vi "Filter Ancestor Names.vi"(8 "error in (no error)":errorcluster, 9 "Name":string, 10 "Start Index":i32, 11 "Config Manager in":refnum<class "Config Manager.lvclass">) -> (0 "error out":errorcluster, 2 "Elements":refnum<class "Config Element.lvclass">[](array[class]), 3 "Config Manager out":refnum<class "Config Manager.lvclass">)   [LabVIEW 2020, in "CDM-Config.lvlib" / "Config Manager.lvclass"]
uses:
  Config Manager.lvclass
  Config Element/Config Element.lvclass
panel:
  out "Array":T1(array[cluster])
  out "delimited string":string
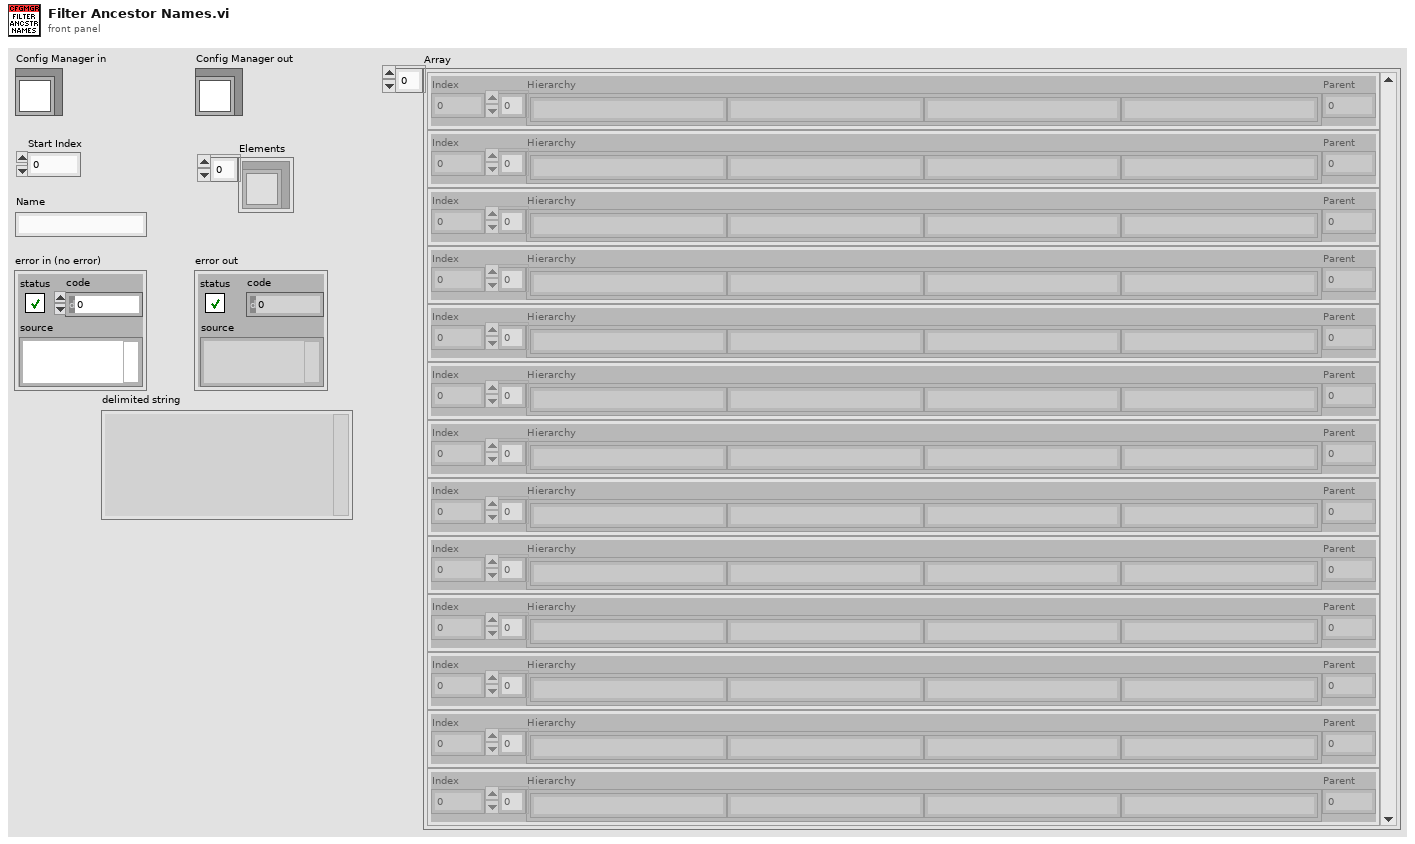
[diagram p1: front panel]
types:
  T1 = cluster{"Index":i32, "Hierarchy":string[], "Parent":i32}[]
  T2 = typedef "CDM-Config.lvlib/Config Manager.lvclass/Ref Data.ctl" = cluster{"Elements":refnum<class "Config Element.lvclass">[], "Hierarchy Map":map{string[], i32}, "Element Map":map{refnum<class "Config Element.lvclass">, i32}}
  T3 = cluster{"Index":i32, "Hierarchy":string[], "Index":i32}
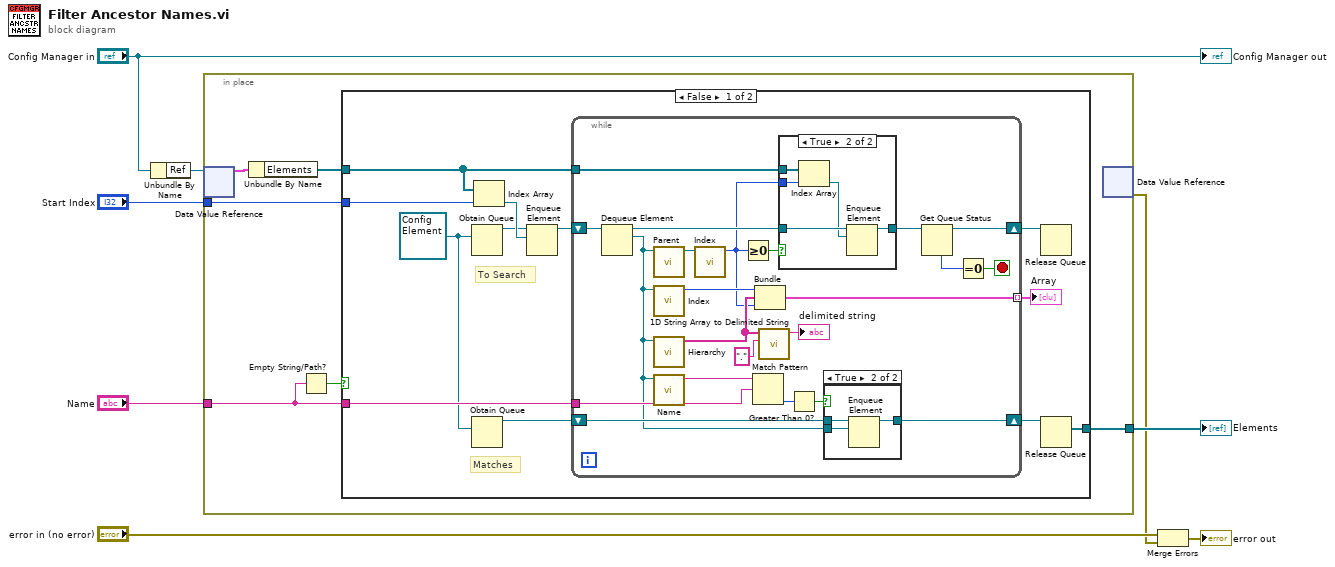
[diagram p0: block diagram]
diagram:
  n1 = Unbundle By Name("Config Manager in") -> ("Ref"=w6:refnum<data-value>)
  n2 = in-place {
    in-place-border: "Start Index" -> [w12]
    in-place-border: "Name" -> [w10]
    in-place-border: [w11] -> w2
    n3 = in-place-dvr #1(w6) -> (w14:T2)  [unwired: 1 out]
    n4 = Unbundle By Name(w14) -> ("Elements"=w13:refnum<class "Config Element.lvclass">[])
    n5 = Empty String/Path?(string/path=w10) -> (empty?=w9:bool)
    n6 = case shown="False" w9 {
      tunnel: w13 -> [w26 w59]
      tunnel: w12 -> [w25 _]
      tunnel: w10 -> [w22 _]
      tunnel: [w16 w59] -> w11
      frame False {
        w21 = refnum<class "Config Element.lvclass"> refnum ("CDM-Config.lvlib:Config Element.lvclass")
        # "Matches"
        # "To Search"
        n7 = Obtain Queue(element data type=w21) -> (queue out=w20:refnum<queue>)  [unwired: 4 in, 2 out]
        n8 = Obtain Queue(element data type=w21) -> (queue out=w19:refnum<queue>)  [unwired: 4 in, 2 out]
        n9 = Index Array(array=w26, index=w25) -> (element=w24:refnum<class "Config Element.lvclass">)
        n10 = Enqueue Element(queue=w20, element=w24) -> (queue out=w23:refnum<queue>)  [unwired: 2 in, 2 out]
        n11 = while {
          tunnel: w26 -> [w41]
          shift-right: [w38] -> w17
          shift-left: w23 -> [w48]
          shift-right: [w42] -> w18
          shift-left: w19 -> [w43]
          tunnel: w22 -> [w46]
          tunnel: [w32] -> w15 mode=indexing
          stop <- w36 stop-if-true
          n12 = Dequeue Element(queue=w48) -> (queue out=w40:refnum<queue>, element=w31:refnum<class "Config Element.lvclass">)  [unwired: 2 in, 2 out]
          n13 = call "Parent.vi"("Config Element in"=w31) -> ("Parent"=w33:refnum<class "Config Element.lvclass">)  [unwired: 9 in, 1 out]
          n14 = call "Index.vi"("Config Element in"=w31) -> ("Index"=w29:i32)  [unwired: 9 in, 1 out]
          n15 = call "Hierarchy.vi"("Config Element in"=w31) -> ("Hierarchy"=w30:string[])  [unwired: 9 in, 1 out]
          n16 = call "Name.vi"("Config Element in"=w31) -> ("Name"=w47:string)  [unwired: 9 in, 1 out]
          n17 = call "Index.vi"("Config Element in"=w33) -> ("Index"=w28:i32)  [unwired: 9 in, 1 out]
          n18 = Greater Or Equal To 0?(x=w28) -> (x >= 0?=w27:bool)
          n19 = Match Pattern(string=w47, regular expression=w46) -> (offset past match=w45:i32)  [unwired: 1 in, 3 out]
          n20 = Bundle("Index"=w29, "Hierarchy"=w30, "Index"=w28) -> (w32:T3)  [unwired: 1 in]
          n21 = call <vilib>:"1D String Array to Delimited String.vi"("delimiter"=".", "string array"=w30) -> ("delimited string"=→"delimited string":string)  [unwired: 9 in]
          n22 = case shown="True" w27 {
            tunnel: w41 -> [_ w54]
            tunnel: w40 -> [w49 w53]
            tunnel: [w49 w52] -> w39
            tunnel: w28 -> [_ w50]
            frame False {
            }
            frame True {
              n23 = Index Array(array=w54, index=w50) -> (element=w51:refnum<class "Config Element.lvclass">)
              n24 = Enqueue Element(queue=w53, element=w51) -> (queue out=w52:refnum<queue>)  [unwired: 2 in, 2 out]
            }
          }
          n25 = Greater Than 0?(x=w45) -> (x > 0?=w44:bool)
          n26 = case shown="True" w44 {
            tunnel: w43 -> [w55 w58]
            tunnel: w31 -> [_ w57]
            tunnel: [w55 w56] -> w42
            frame False {
            }
            frame True {
              n27 = Enqueue Element(queue=w58, element=w57) -> (queue out=w56:refnum<queue>)  [unwired: 2 in, 2 out]
            }
          }
          n28 = Get Queue Status(queue=w39) -> (queue out=w38:refnum<queue>, # elements in queue=w37:i32)  [unwired: 2 in, 6 out]
          n29 = Equal To 0?(x=w37) -> (x = 0?=w36:bool)
        }
        "Array" <- w15
        n30 = Release Queue(queue=w17) -> ()  [unwired: 2 in, 3 out]
        n31 = Release Queue(queue=w18) -> (remaining elements=w16:refnum<class "Config Element.lvclass">[])  [unwired: 2 in, 2 out]
      }
      frame True {
      }
    }
    n32 = in-place-dvr #1() -> (w1:errorcluster)  [unwired: 1 in, 1 out]
  }
  "Elements" <- w2
  n33 = Merge Errors("error in (no error)", w1) -> (→"error out":errorcluster)
  "Config Manager out" <- "Config Manager in"
